vi "Main.vi"(11 "Module Admin":refnum<class "Delacor_lib_QMH_Module Admin.lvclass">) -> ()   [LabVIEW 2021, in "RT Main.lvlib"]
doc: "This template is based off of the Queued Message Handler design pattern and the Queued Message Handler project template that ships with LabVIEW.\n\nThe main difference is that the queue is private to this module and communication between modules is performed via Broadcast and Request events.\n\nRequest events are wrapped in public API methods and are handled in the Event Handling Loop (EHL) of this VI. Any module can register for Broadcast events sent by this module. The EHL generates messages based on user interface actions.\n\nThe Message Handling Loop (MHL) processes messages generated by the EHL, or by other messages. The messages are string values, so new messages can be added easily to the Message Cases case structure in the MHL. Each message cluster can also provide an optional value for Message Data, which is a variant that can be converted to whatever message-specific data is required.\n_____\nBased on DQMH Dev Tools: Project Template 7.1.2.1547."
uses:
  RT Main.lvlib
  <vilib>/Delacor/Delacor QMH/Libraries/Module Admin_class/Delacor_lib_QMH_Module Admin.lvclass
  Module Data--cluster.ctl
  <vilib>/myRIO/Instrument Drivers/Onboard IO/AI/typedefs/AI Reference.ctl
  <vilib>/myRIO/Common/Instrument Driver Framework/Utilities/typedefs/myRIO Generic Hardware Reference.ctl
  <vilib>/myRIO/Common/Instrument Driver Framework/Utilities/typedefs/Hardware Version Enum.ctl
  <vilib>/myRIO/Common/Instrument Driver Framework/Utilities/typedefs/myRIO v1.0 Reference.ctl
  <vilib>/myRIO/Common/Instrument Driver Framework/Utilities/typedefs/Generic FPGA Reference.ctl
  <vilib>/myRIO/Common/Instrument Driver Framework/myRIO v1.0/AI/typedefs/AI Channels List.ctl
  <vilib>/myRIO/Common/Instrument Driver Framework/myRIO v1.0/AI/typedefs/AI Channels Enum.ctl
  <vilib>/myRIO/Common/Instrument Driver Framework/Utilities/typedefs/Analog Scaling Constants List.ctl
  <vilib>/myRIO/Common/Instrument Driver Framework/Utilities/typedefs/Analog Scaling Constants.ctl
  <vilib>/myRIO/Instrument Drivers/Onboard IO/DIO/typedefs/DIO Reference.ctl
  <vilib>/myRIO/Common/Instrument Driver Framework/myRIO v1.0/DIO/typedefs/DIO Channels List.ctl
  <vilib>/myRIO/Common/Instrument Driver Framework/myRIO v1.0/DIO/typedefs/DIO Channels Enum.ctl
  Libraries/Common RT/Modules Launched.ctl
  RT FIFOS--cluster.ctl
  Libraries/Common RT/Hardware Monitoring.ctl
  Hardware Monitoring TL--cluster.ctl
  Stop Argument--cluster.ctl
  <vilib>/Delacor/Delacor QMH/Libraries/Message Queue_class/Delacor_lib_QMH_Message Queue.lvclass/Delacor_lib_QMH_Message Queue.ctl
  <vilib>/Delacor/Delacor QMH/Libraries/Module Admin_class/Delacor_lib_QMH_Module Admin.lvclass/Delacor_lib_QMH_Module Admin.ctl
  Create RT FIFOs Argument--cluster.ctl
  Control Loop Cluster.ctl
  Data Cluster.ctl
  <vilib>/Delacor/Delacor QMH/Libraries/Message Queue_class/Delacor_lib_QMH_Enqueue Message (Single).vi
  <vilib>/Delacor/Delacor QMH/Libraries/Module Admin_class/Delacor_lib_QMH_Get External Launch.vi
  <vilib>/nisyscfg/Close (System).vi
  Timed Loop.vi
  <vilib>/Delacor/Delacor QMH/Libraries/Message Queue_class/Delacor_lib_QMH_Message Queue.lvclass
  Analog Input/Analog Input.lvlib
  <vilib>/myRIO/Instrument Drivers/Onboard IO/AI/AI.lvlib
  Libraries/Common RT/Common RT.lvlib
  <vilib>/nisyscfg/nisyscfg.lvlib
  Digital Inputs/Digital Inputs.lvlib
  <vilib>/myRIO/Instrument Drivers/Onboard IO/DIO/DIO.lvlib
  TDMS/TDMS.lvlib
  RT Interpreter/Manager/RT Interpreter Manager.lvlib
panel:
  out "error out 3":errorcluster
  out "error out 2":errorcluster
  out "error out":errorcluster
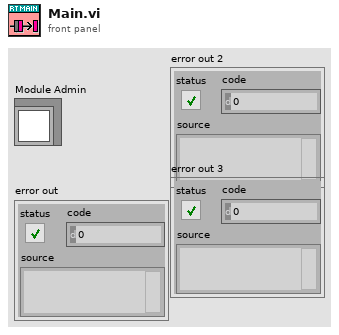
[diagram p1: front panel]
types:
  T1 = typedef "RT Main.lvlib/Request Events--cluster.ctl" = cluster{"Stop Module":refnum<user-event>, "Show Panel":refnum<user-event>, "Hide Panel":refnum<user-event>, "Get Module Execution Status":refnum<user-event>, "Show Diagram":refnum<user-event>, "Private.Launch Control Loop":refnum<user-event>, "Private.RT FIFO Ref":refnum<user-event>, "Private.Create RT FIFOs":refnum<user-event>}
  T2 = typedef "Analog Input.lvlib/Broadcast Events--cluster.ctl" = cluster{"Module Did Init":refnum<user-event>, "Status Updated":refnum<user-event>, "Error Reported":refnum<user-event>, "Module Did Stop":refnum<user-event>, "Update Module Execution Status":refnum<user-event>, "AI Input Reference":refnum<user-event>}
  T3 = typedef "Digital Inputs.lvlib/Broadcast Events--cluster.ctl" = cluster{"Module Did Init":refnum<user-event>, "Status Updated":refnum<user-event>, "Error Reported":refnum<user-event>, "Module Did Stop":refnum<user-event>, "Update Module Execution Status":refnum<user-event>, "Send DI Reference":refnum<user-event>}
  T4 = typedef "TDMS.lvlib/Broadcast Events--cluster.ctl" = cluster{"Module Did Init":refnum<user-event>, "Status Updated":refnum<user-event>, "Error Reported":refnum<user-event>, "Module Did Stop":refnum<user-event>, "Update Module Execution Status":refnum<user-event>}
  T5 = typedef "RT Interpreter Manager.lvlib/Broadcast Events--cluster.ctl" = cluster{"Module Did Init":refnum<user-event>, "Status Updated":refnum<user-event>, "Error Reported":refnum<user-event>, "Module Did Stop":refnum<user-event>, "Update Module Execution Status":refnum<user-event>}
  T6 = typedef "RT Main.lvlib/Hardware Monitoring TL--cluster.ctl" = cluster{"Session in":refnum<k21>, "RT FIFOs--cluster":T7}
  T7 = typedef "RT Main.lvlib/RT FIFOS--cluster.ctl" = cluster{"AIs RT FIFO out":refnum<k33>, "DIOs RT FIFO out":refnum<k33>, "System Status RT FIFO":refnum<k33>}
  T8 = typedef "RT Main.lvlib/Module Data--cluster.ctl" = cluster{"Status":string, "Current Directory":path, "AI Reference":T9, "DIO Reference":T18, "Modules Launched":T21, "RT FIFOs--cluster":T7}
  T9 = typedef "AI.lvlib/AI Reference.ctl" = cluster{"myRIO Reference":T10, "AI Channels List":T14, "AI Scaling Constants List":T16}
  T10 = typedef "myRIO Generic Hardware Reference.ctl" = cluster{"myRIO Model":T11, "myRIO Hardware Reference":T12}
  T11 = typedef "Hardware Version Enum.ctl" = enum16{"Unknown", "myRIO-1900", "myRIO-1950", "roboRIO", "NI ELVIS RIO CM", "ELVIS III"}
  T12 = typedef "myRIO v1.0 Reference.ctl" = cluster{"Generic FPGA Reference":T13, "Allow multiple opens":bool}
  T13 = typedef "Generic FPGA Reference.ctl" = refnum<k20>
  T14 = typedef "AI Channels List.ctl" = T15[]
  T15 = typedef "AI Channels Enum.ctl" = enum16{"Not Connected", "AudioIn/Left", "AudioIn/Right", "C/AI0", "C/AI1", "A/AI0", "A/AI1", "A/AI2", "A/AI3", "A/AI4", "A/AI5", "A/AI6", "A/AI7", "B/AI0", "B/AI1", "B/AI2", "B/AI3", "B/AI4", "B/AI5", "B/AI6", "B/AI7", "AI/AI0", "AI/AI1", "AI/AI2", "AI/AI3", "A/AI0 (DIFF)", "A/AI1 (DIFF)", "A/AI2 (DIFF)", "A/AI3 (DIFF)", "B/AI0 (DIFF)", "B/AI1 (DIFF)", "B/AI2 (DIFF)", "B/AI3 (DIFF)"}
  T16 = typedef "Analog Scaling Constants List.ctl" = T17[]
  T17 = typedef "Analog Scaling Constants.ctl" = cluster{"LSB Weight (Volts)":dbl, "Offset (Volts)":dbl, "Signed?":bool}
  T18 = typedef "DIO.lvlib/DIO Reference.ctl" = cluster{"myRIO Reference":T10, "DIO Channels List":T19}
  T19 = typedef "DIO Channels List.ctl" = T20[]
  T20 = typedef "DIO Channels Enum.ctl" = enum16{"Not Connected", "C/DIO0", "C/DIO1", "C/DIO2", "C/DIO3", "C/DIO4", "C/DIO5", "C/DIO6", "C/DIO7", "A/DIO0", "A/DIO1", "A/DIO2", "A/DIO3", "A/DIO4", "A/DIO5", "A/DIO6", "A/DIO7", "A/DIO8", "A/DIO9", "A/DIO10", "A/DIO11", "A/DIO12", "A/DIO13", "A/DIO14", "A/DIO15", "A/DIO16", "A/DIO17", "A/DIO18", "A/DIO19", "B/DIO0", "B/DIO1", "B/DIO2", "B/DIO3", "B/DIO4", "B/DIO5", "B/DIO6", "B/DIO7", "B/DIO8", "B/DIO9", "B/DIO10", "B/DIO11", "B/DIO12", "B/DIO13", "B/DIO14", "B/DIO15", "B/DIO16", "B/DIO17", "B/DIO18", "B/DIO19", "LED0", "LED1", "LED2", "LED3", "Button0", "DIO/DIO0", "DIO/DIO1", "DIO/DIO2", "DIO/DIO3", "DIO/DIO4", "DIO/DIO5", "DIO/DIO6", "DIO/DIO7", "DIO/DIO8", "DIO/DIO9", "SPI/CS0", "SPI/CS1", "SPI/CS2", "SPI/CS3", "LED RADIO (Green)", "LED RADIO (Red)", "LED COMM (Green)", "LED COMM (Red)", "LED MODE (Green)", "LED MODE (Red)"}
  T21 = typedef "Common RT.lvlib/Modules Launched.ctl" = cluster{"AI Input":bool, "DI Input":bool, "TDMS Module":bool, "UDP Module":bool}
  T22 = enum32{"invalid lock state", "Not Locked", "Locked (No Password)", "Password-protected"}
  T23 = typedef "RT Main.lvlib/Stop Argument--cluster.ctl" = cluster{"Origin":string, "Exit via Stop Module Req?":bool, "Wait for Module to stop?":bool}
  T24 = typedef "RT Main.lvlib/Create RT FIFOs Argument--cluster.ctl" = cluster{"Boolean":bool}
  T25 = typedef "RT Main.lvlib/Control Loop Cluster.ctl" = cluster{"AI Reference":T9, "DIO Reference":T18, "Data Cluster":T26, "TDMS Record?":bool, "Writing?":bool, "RT FIFOs--cluster":T7}
  T26 = typedef "RT Main.lvlib/Data Cluster.ctl" = cluster{"Analog Input":dbl[], "Digital Inputs":bool[], "System Status":T27, "Iteration Duration (ms)":dbl, "Finish Late?":bool}
  T27 = typedef "Common RT.lvlib/Hardware Monitoring.ctl" = cluster{"Memory RAM Free (%)":dbl, "Free Flash memory (%)":dbl, "CPU 0 (%)":u32, "CPU 1 (%)":u32}
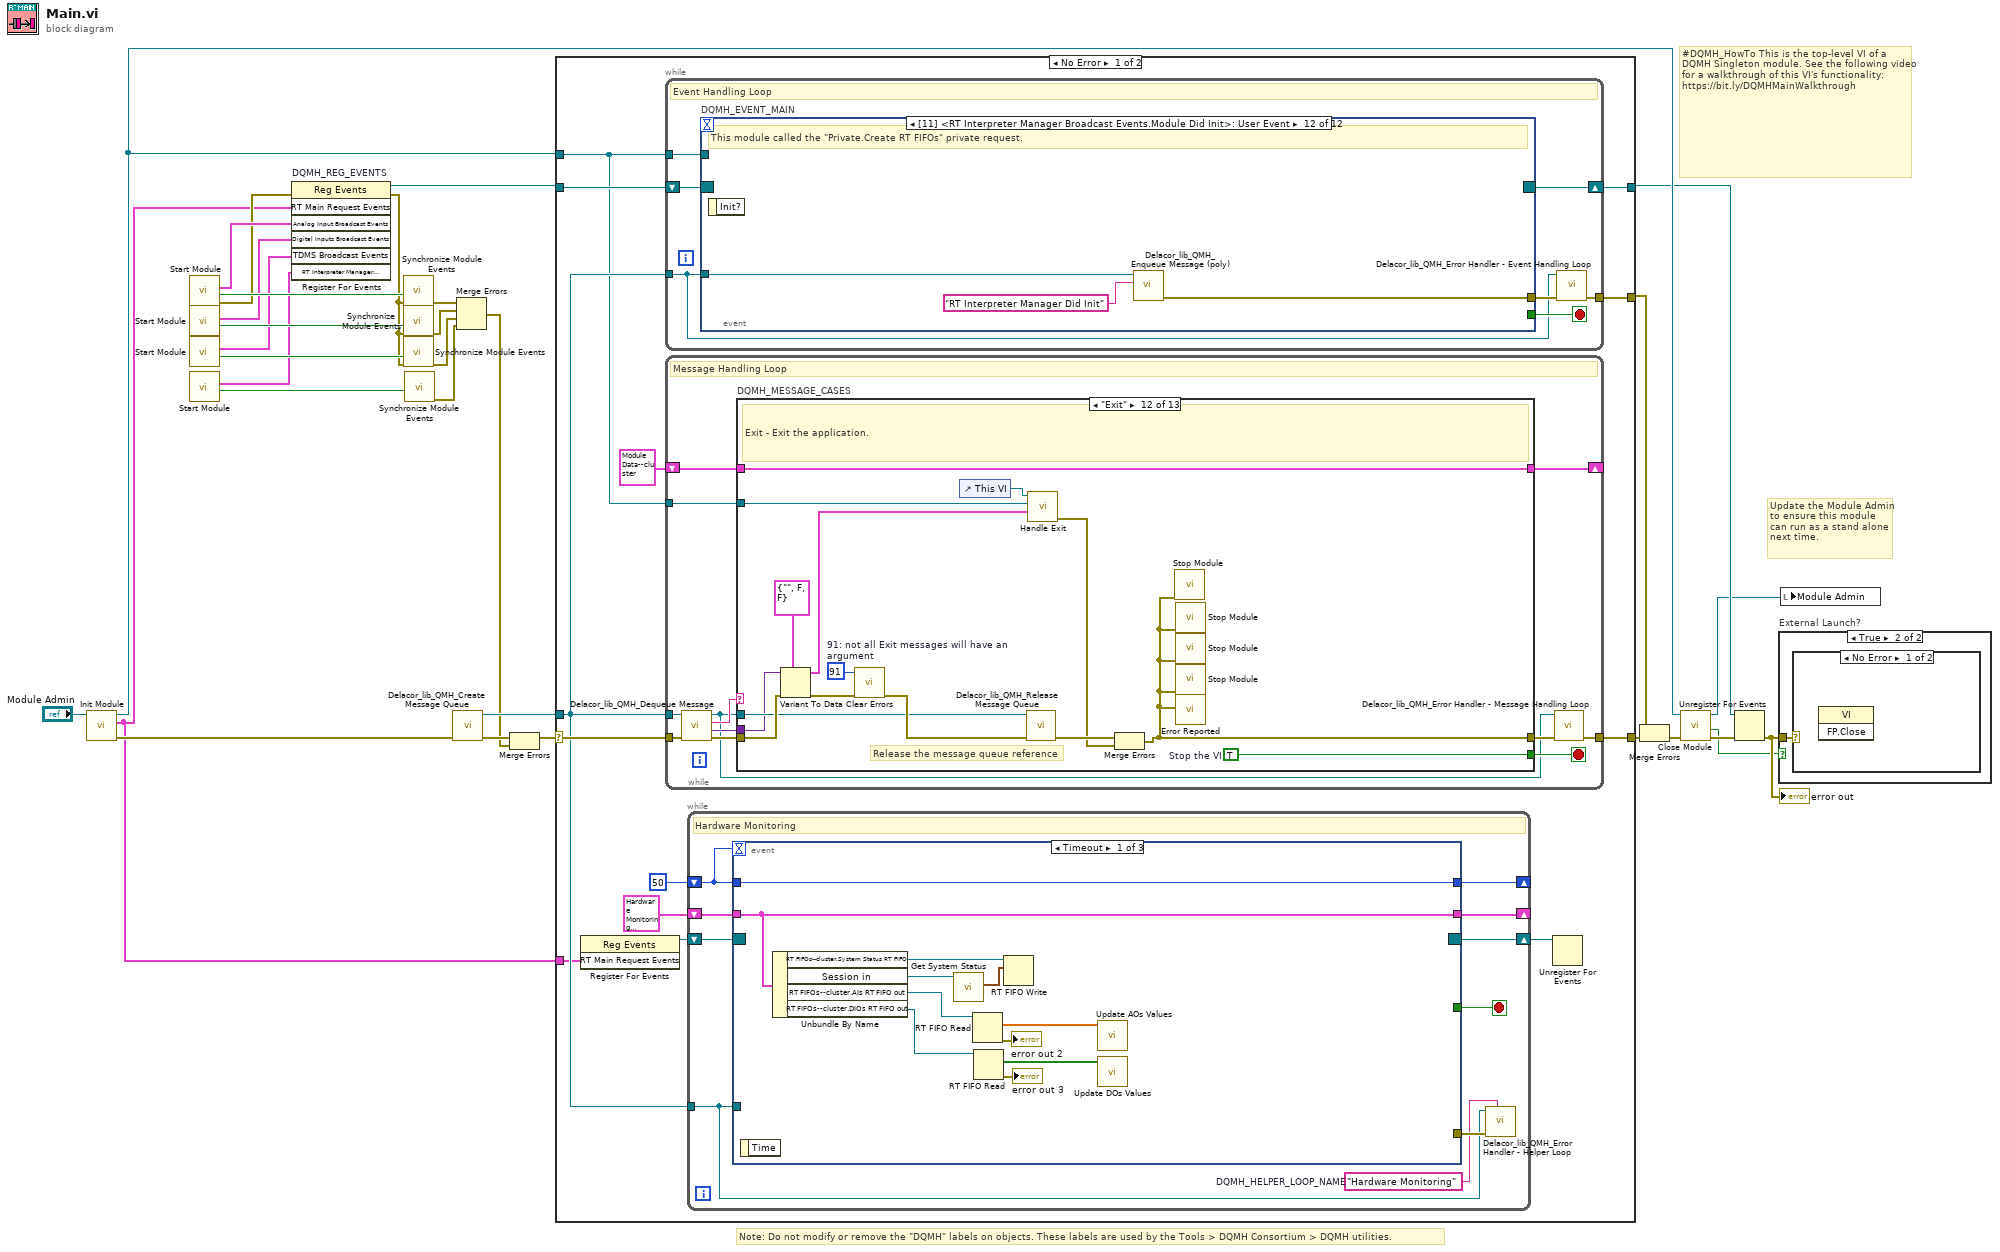
[diagram p0: block diagram]
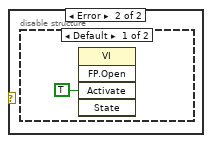
[diagram p3: hidden frame]
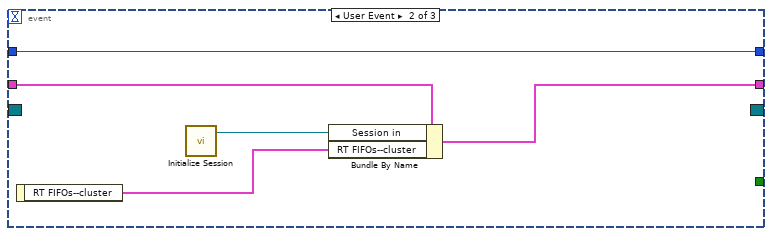
[diagram p5: hidden frame]
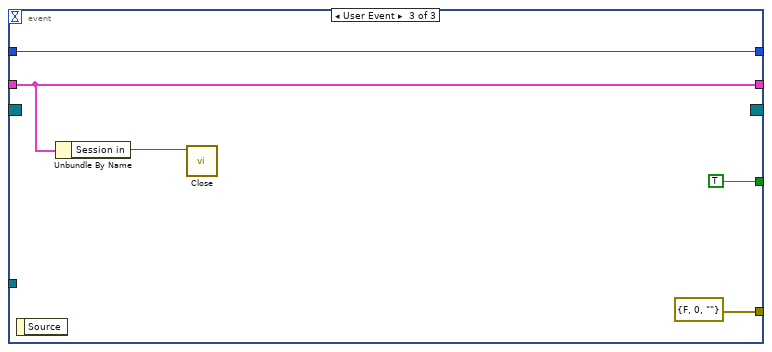
[diagram p6: hidden frame]
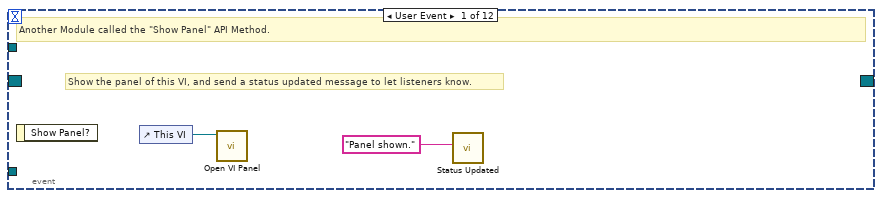
[diagram p7: hidden frame]
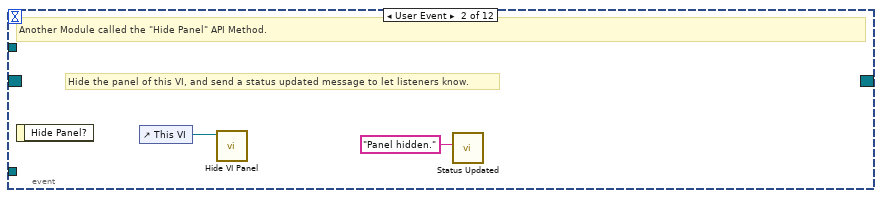
[diagram p8: hidden frame]
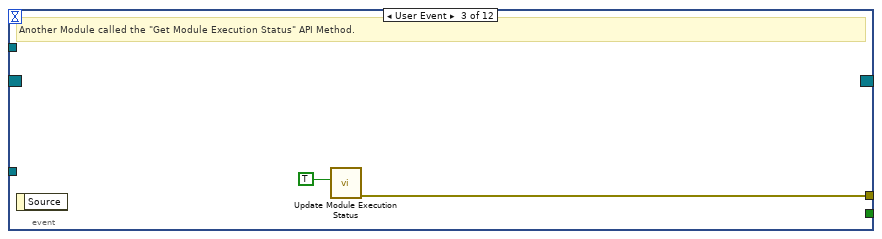
[diagram p9: hidden frame]
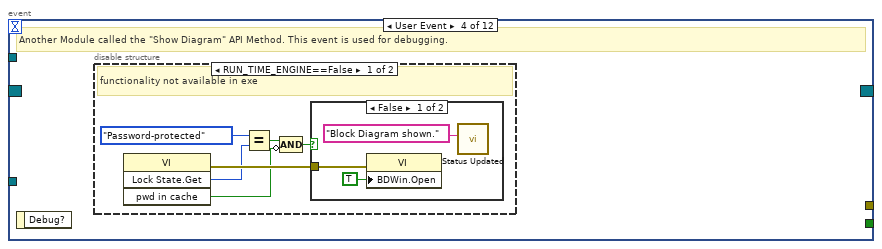
[diagram p10: hidden frame]
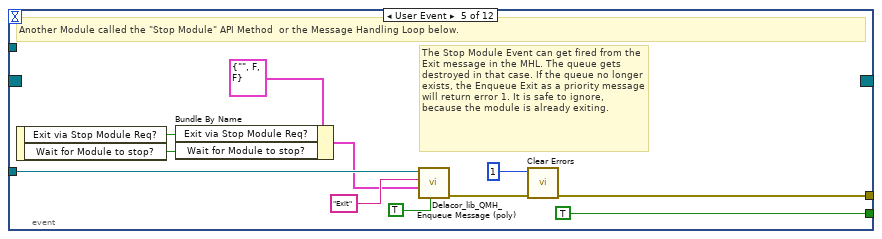
[diagram p13: hidden frame]
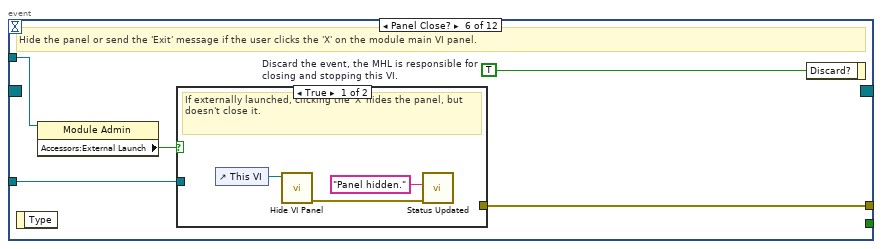
[diagram p14: hidden frame]
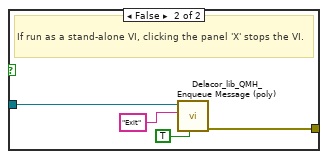
[diagram p15: hidden frame]
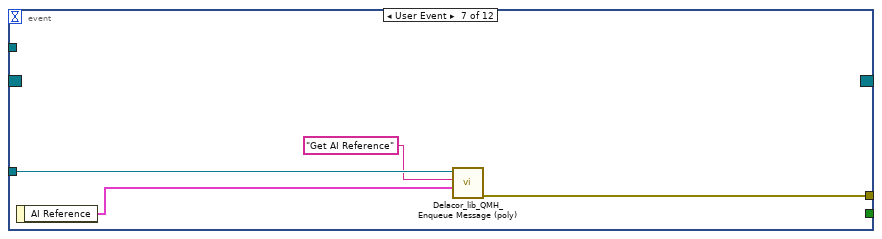
[diagram p16: hidden frame]
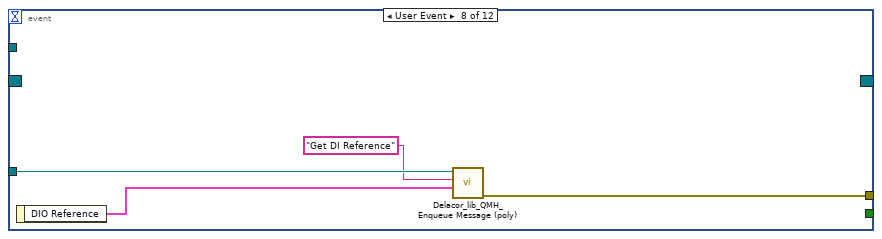
[diagram p17: hidden frame]
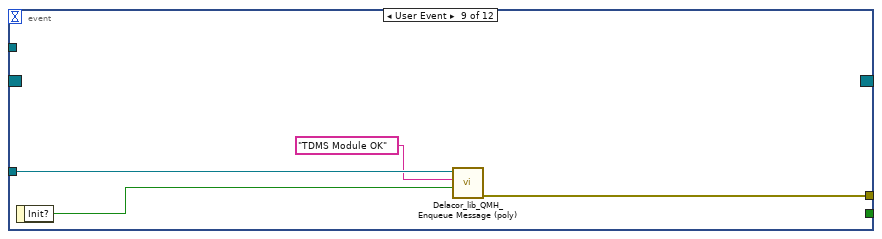
[diagram p18: hidden frame]
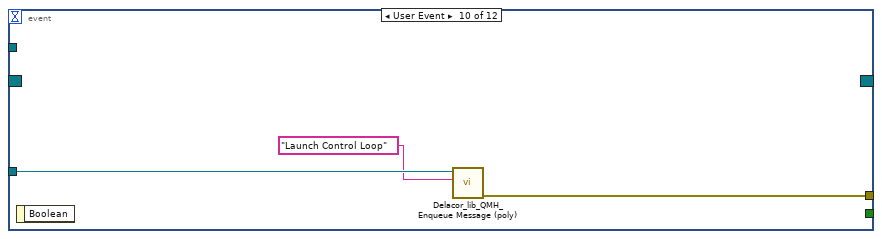
[diagram p19: hidden frame]
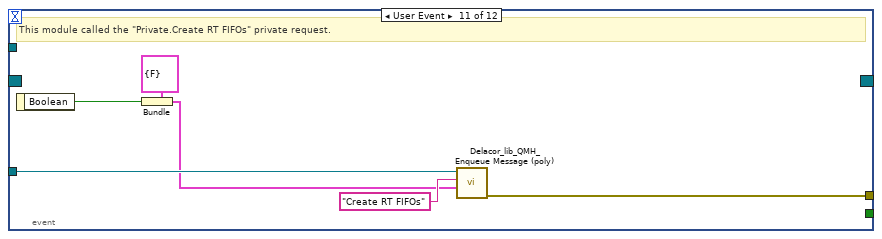
[diagram p20: hidden frame]
diagram:
  # "#DQMH_HowTo This is the top-level VI of a DQMH Singleton module. See the following video for a walkthrough of this VI's functionality: https://bit.ly/DQMHMainWalkthrough"
  # "Note: Do not modify or remove the \"DQMH\" labels on objects. These labels are used by the Tools > DQMH Consortium > DQMH utilities."
  # "Update the Module Admin to ensure this module can run as a stand alone next time."
  n1 = call "Init Module.vi"("Singleton Module Admin in"="Module Admin") -> ("error out"=w30:errorcluster, "RT Main Request Events"=w11:T1, "Singleton Module Admin out"=w23:refnum<class "Delacor_lib_QMH_Module Admin.lvclass">)  [unwired: 8 in]
  n2 = call "Start Module.vi"() -> ("error out"=w14:errorcluster, "Wait for Event Sync?"=w15:bool, "Analog Input Broadcast Events"=w16:T2)  [unwired: 7 in, 2 out]
  n3 = call "Start Module.vi"() -> ("Wait for Event Sync?"=w10:bool, "Digital Inputs Broadcast Events"=w9:T3)  [unwired: 7 in, 3 out]
  n4 = call "Start Module.vi"() -> ("Wait for Event Sync?"=w6:bool, "TDMS Broadcast Events"=w7:T4)  [unwired: 8 in, 2 out]
  n5 = call "Start Module.vi"() -> ("Wait for Event Sync?"=w1:bool, "RT Interpreter Manager Broadcast Events"=w2:T5)  [unwired: 7 in, 3 out]
  n6 = register-events "DQMH_REG_EVENTS"(error in=w14, w11, w16, w9, w7, w2) -> (reference out=w21:refnum<event-registration>, error out=w4:errorcluster)  [unwired: 1 in]
  n7 = call "Synchronize Module Events.vi"("error in"=w4, "Wait for Event Sync?"=w15) -> ("error out"=w13:errorcluster)  [unwired: 9 in]
  n8 = call "Synchronize Module Events.vi"("error in"=w4, "Wait for Event Sync?"=w10) -> ("error out"=w8:errorcluster)  [unwired: 9 in]
  n9 = call "Synchronize Module Events.vi"("error in"=w4, "Wait for Event Sync?"=w6) -> ("error out"=w5:errorcluster)  [unwired: 9 in]
  n10 = call "Synchronize Module Events.vi"("Wait for Event Sync?"=w1) -> ("error out"=w3:errorcluster)  [unwired: 10 in]
  n11 = call <vilib>:"Delacor_lib_QMH_Create Message Queue.vi"("error in"=w30) -> ("error out"=w25:errorcluster, "Message Queue"=w20:refnum<class "Delacor_lib_QMH_Message Queue.lvclass">)  [unwired: 9 in]
  n12 = Merge Errors(w13, w8, w5, w3) -> (w12:errorcluster)
  n13 = Merge Errors(w25, w12) -> (w24:errorcluster)
  n14 = case shown="No Error" w24 {
    selector: w24 -> [w42 w296]
    tunnel: [w44 w295] -> w31
    tunnel: [w41 w294] -> w22
    tunnel: w21 -> [w39 w294]
    tunnel: w20 -> [w38 w289]
    tunnel: [w43 _] -> w28
    tunnel: w23 -> [w37 w290]
    tunnel: w11 -> [w36 _]
    frame No Error {
      n15 = register-events ("DQMH_HELPER_REGFOREVENTS")(w36) -> (reference out=w34:refnum<event-registration>)  [unwired: 2 in, 1 out]
      n16 = while {
        tunnel: w38 -> [w76]
        shift-right: [w79] -> w41
        shift-left: w39 -> [w80]
        tunnel: [w81] -> w43
        tunnel: w37 -> [w77]
        stop <- w78 stop-if-true
        # "Event Handling Loop"
        n17 = event "DQMH_EVENT_MAIN" shown="[11] <RT Interpreter Manager Broadcast Events.Module Did Init>: User Event" {
          selector: w80 -> [_ _ _ _ _ _ _ _ _ _ _ _]
          dyn-events: [_ _ _ _ _ _ _ _ _ _ _ _] -> w79
          timeout: _ -> [_ _ _ _ _ _ _ _ _ _ _ _]
          tunnel: [_ _ _ _ TRUE ("Discard?") _ _ _ _ _ _ _] -> w78
          tunnel: w76 -> [_ _ _ _ w104 w111 w124 w128 w132 w135 w141 w144]
          tunnel: [_ _ w88 _ w107 w113 w121 w125 w129 w133 w136 w142] -> w82
          tunnel: w77 -> [_ _ _ _ _ w110 _ _ _ _ _ _]
          event User Event {
            # "Show the panel of this VI, and send a status updated message to let listeners know."
            # "Another Module called the \"Show Panel\" API Method."
            n18 = event-data() -> ()  [unwired: 1 in, 1 out]
            n19 = control-ref of="This VI"() -> (w84:refnum<vi>)
            n20 = call "Open VI Panel.vi"("VI"=w84) -> ()  [unwired: 10 in, 1 out]
            n21 = call "Status Updated.vi"("Status"="Panel shown." ("format string")) -> ()  [unwired: 10 in, 1 out]
          }
          event User Event {
            # "Hide the panel of this VI, and send a status updated message to let listeners know."
            # "Another Module called the \"Hide Panel\" API Method."
            n22 = event-data() -> ()  [unwired: 1 in, 1 out]
            n23 = control-ref of="This VI"() -> (w86:refnum<vi>)
            n24 = call "Hide VI Panel.vi"("VI"=w86) -> ()  [unwired: 10 in, 1 out]
            n25 = call "Status Updated.vi"("Status"="Panel hidden." ("format string")) -> ()  [unwired: 10 in, 1 out]
          }
          event User Event {
            # "Another Module called the \"Get Module Execution Status\" API Method."
            n26 = event-data() -> ()  [unwired: 1 in, 1 out]
            n27 = call "Update Module Execution Status.vi"("Running?"=TRUE) -> ("error out"=w88:errorcluster)  [unwired: 10 in]
          }
          event User Event {
            # "Another Module called the \"Show Diagram\" API Method. This event is used for debugging."
            n28 = event-data() -> ()  [unwired: 1 in, 1 out]
            n29 = disable-structure shown="RUN_TIME_ENGINE==False" {
              frame condition #0 (active) {
                # "functionality not available in exe"
                n30 = invoke on="Invoke Node" class="VI" method="Lock State.Get"() -> (error out=w94:errorcluster, "Get Lock State"=w93:T22, "pwd in cache"=w90:bool)  [unwired: 4 in, 1 out]
                n31 = Equal?(x=T22."Password-protected", y=w93) -> (x = y?=w91:bool)
                n32 = Compound Arithmetic op=AND(w91, invert w90) -> (w89:bool)
                n33 = case shown="False" w89 {
                  tunnel: w94 -> [w97 _]
                  frame False {
                    n34 = property on="Property Node" class="VI"(error in=w97, "BDWin.Open"=TRUE ("Block Diagram Window:Open")) -> ()  [unwired: 1 in, 2 out]
                    n35 = call "Status Updated.vi"("Status"="Block Diagram shown." ("format string")) -> ()  [unwired: 10 in, 1 out]
                  }
                  frame True {
                    # "Password-protected VI, and the password is not in the cache. Do not show the diagram."
                  }
                }
              }
              frame condition #1 {
              }
            }
          }
          event User Event {
            # "The Stop Module Event can get fired from the Exit message in the MHL. The queue gets destroyed in that case. If the queue no longer exists, the Enqueue Exit as a priority message will return error 1. It is safe to ignore, because the module is already exiting."
            # "Another Module called the \"Stop Module\" API Method  or the Message Handling Loop below."
            n36 = event-data() -> ("Exit via Stop Module Req?"=w100:bool, "Wait for Module to stop?"=w99:bool)  [unwired: 1 in]
            n37 = Bundle By Name(cluster=T23 {"Origin"="", "Exit via Stop Module Req?"=FALSE, "Wait for Module to stop?"=FALSE} ("Stop Argument"), "Exit via Stop Module Req?"=w100, "Wait for Module to stop?"=w99) -> (w98:T23)
            n38 = call-poly <vilib>:"Delacor_lib_QMH_Enqueue Message (poly).vi"("Priority Message? (F)"=TRUE, "Message Data"=w98, "Message"="Exit", "Message Queue in"=w104) -> ("error out"=w108:errorcluster)  [unwired: 6 in, 1 out]
            n39 = call <vilib>:"Clear Errors.vi"("error in (no error)"=w108, "specific error code to clear (0: all)"=1) -> ("error out"=w107:errorcluster)  [unwired: 4 in, 1 out]
          }
          event Panel Close? {
            w112 = TRUE  # Discard the event, the MHL is responsible for closing and stopping this VI.
            # "Hide the panel or send the 'Exit' message if the user clicks the 'X' on the module main VI panel."
            n40 = event-data() -> ()  [unwired: 1 in, 1 out]
            n41 = property on="Property Node" class="Module Admin"(reference=w110) -> ("Accessors:External Launch"=w109:bool)  [unwired: 1 in, 2 out]
            n42 = case shown="True" w109 {
              tunnel: w111 -> [_ w119]
              tunnel: [_ w120] -> w113
              frame True {
                # "If externally launched, clicking the 'X' hides the panel, but doesn't close it."
                n43 = control-ref of="This VI"() -> (w116:refnum<vi>)
                n44 = call "Hide VI Panel.vi"("VI"=w116) -> ("error out"=w114:errorcluster)  [unwired: 10 in]
                n45 = call "Status Updated.vi"("error in"=w114, "Status"="Panel hidden." ("format string")) -> ()  [unwired: 9 in, 1 out]
              }
              frame False {
                # "If run as a stand-alone VI, clicking the panel 'X' stops the VI."
                n46 = call-poly <vilib>:"Delacor_lib_QMH_Enqueue Message (poly).vi"("Priority Message? (F)"=TRUE, "Message"="Exit", "Message Queue in"=w119) -> ("error out"=w120:errorcluster)  [unwired: 7 in, 1 out]
              }
            }
            n47 = event-data ("Event Filter Node")("Discard?"=w112) -> ()  [unwired: 1 in, 1 out]
          }
          event User Event {
            n48 = event-data() -> ("AI Reference"=w122:T9)  [unwired: 1 in]
            n49 = call-poly <vilib>:"Delacor_lib_QMH_Enqueue Message (poly).vi"("Message Data"=w122, "Message"="Get AI Reference", "Message Queue in"=w124) -> ("error out"=w121:errorcluster)  [unwired: 7 in, 1 out]
          }
          event User Event {
            n50 = event-data() -> ("DIO Reference"=w126:T18)  [unwired: 1 in]
            n51 = call-poly <vilib>:"Delacor_lib_QMH_Enqueue Message (poly).vi"("Message Data"=w126, "Message"="Get DI Reference", "Message Queue in"=w128) -> ("error out"=w125:errorcluster)  [unwired: 7 in, 1 out]
          }
          event User Event {
            n52 = event-data() -> ("Init?"=w130:bool)  [unwired: 1 in]
            n53 = call-poly <vilib>:"Delacor_lib_QMH_Enqueue Message (poly).vi"("Message Data"=w130, "Message"="TDMS Module OK", "Message Queue in"=w132) -> ("error out"=w129:errorcluster)  [unwired: 7 in, 1 out]
          }
          event User Event {
            n54 = event-data() -> ()  [unwired: 1 in, 1 out]
            n55 = call-poly <vilib>:"Delacor_lib_QMH_Enqueue Message (poly).vi"("Message"="Launch Control Loop", "Message Queue in"=w135) -> ("error out"=w133:errorcluster)  [unwired: 8 in, 1 out]
          }
          event User Event {
            # "This module called the \"Private.Create RT FIFOs\" private request."
            n56 = event-data() -> ("Boolean"=w137:bool)  [unwired: 1 in]
            n57 = Bundle(cluster=T24 {"Boolean"=FALSE} ("Create RT FIFOs Argument"), "Boolean"=w137) -> (w138:T24)
            n58 = call-poly <vilib>:"Delacor_lib_QMH_Enqueue Message (poly).vi"("Message Data"=w138, "Message"="Create RT FIFOs", "Message Queue in"=w141) -> ("error out"=w136:errorcluster)  [unwired: 7 in, 1 out]
          }
          event User Event {
            # "This module called the \"Private.Create RT FIFOs\" private request."
            n59 = event-data() -> ()  [unwired: 1 in, 1 out]
            n60 = call-poly <vilib>:"Delacor_lib_QMH_Enqueue Message (poly).vi"("Message"="RT Interpreter Manager Did Init", "Message Queue in"=w144) -> ("error out"=w142:errorcluster)  [unwired: 8 in, 1 out]
          }
        }
        n61 = call-dynamic "Delacor_lib_QMH_Error Handler - Event Handling Loop.vi"("error in"=w82, "Message Queue in"=w76) -> ("dup error in"=w81:errorcluster)  [unwired: 8 in, 1 out]
      }
      n62 = while {
        tunnel: w38 -> [w145]
        shift-right: [w153] -> _
        shift-left: T8 {"Status"="", "Current Directory"=path "", "AI Reference"={"myRIO Reference"={"myRIO Model"=enum."Unknown", "myRIO Hardware Reference"={"Generic FPGA Reference"=refnum, "Allow multiple opens"=FALSE}}, "AI Channels List"=[], "AI Scaling Constants List"=[]}, "DIO Reference"={"myRIO Reference"={"myRIO Model"=enum."Unknown", "myRIO Hardware Reference"={"Generic FPGA Reference"=refnum, "Allow multiple opens"=FALSE}}, "DIO Channels List"=[]}, "Modules Launched"={"AI Input"=FALSE, "DI Input"=FALSE, "TDMS Module"=FALSE, "UDP Module"=FALSE}, "RT FIFOs--cluster"={"AIs RT FIFO out"=refnum, "DIOs RT FIFO out"=refnum, "System Status RT FIFO"=refnum}} ("Data Cluster") -> [w154]
        tunnel: w42 -> [w156]
        tunnel: [w148] -> w44
        tunnel: w37 -> [w149]
        stop <- w152 stop-if-true
        # "Message Handling Loop"
        n63 = call-dynamic "Delacor_lib_QMH_Dequeue Message.vi"("error in"=w156, "Message Queue in"=w145) -> ("error out"=w155:errorcluster, "Message Data"=w150:variant, "Message"=w151:string, "Message Queue out"=w146:refnum<class "Delacor_lib_QMH_Message Queue.lvclass">)  [unwired: 6 in]
        n64 = case "DQMH_MESSAGE_CASES" shown="\"Exit\"" w151 {
          selector: w151 -> [_ _ _ _ _ _ _ _ _ _ _ _ w284]
          tunnel: w146 -> [_ _ _ _ _ _ _ _ _ _ w250 w273 _]
          tunnel: w155 -> [w167 w169 w181 w196 w207 w218 w229 w240 w244 w246 w257 w278 w287]
          tunnel: [w158 w169 w170 w187 w200 w211 w230 w237 w243 w246 w253 w264 w288] -> w147
          tunnel: w154 -> [w159 w168 w176 w193 w205 w216 w235 w241 w242 w245 w252 w272 w285]
          tunnel: [w160 w168 w175 w192 w204 w215 w235 w238 w242 w245 w252 w272 w285] -> w153
          tunnel: [_ _ _ _ _ _ _ _ _ _ _ w271 _] -> w152
          tunnel: w150 -> [_ _ w180 w195 _ _ _ _ _ _ w251 w270 _]
          tunnel: w149 -> [w165 _ _ _ _ _ _ _ _ _ w249 w265 _]
          frame "Initialize" {
            # "Initialize - Any operation that needs to be done before the module can receive messages. Synchronize Caller Events.vi will inform Start Module.vi that the module has launched and is ready to receive messages. Module Did Init.vi will broadcast that the module initialized."
            n65 = call "Synchronize Caller Events.vi"("error in"=w167, "Singleton Module Admin in"=w165) -> ("error out"=w166:errorcluster)  [unwired: 8 in, 1 out]
            n66 = call "Module Name--constant.vi"() -> ("Module Name"=w163:string)  [unwired: 11 in]
            n67 = call "Module Did Init.vi"("error in"=w166, "Initialized?"=TRUE, "Origin"=w163) -> ("error out"=w157:errorcluster)  [unwired: 8 in]
            n68 = Current VI's Path() -> (path=w162:path)
            n69 = Strip Path(path=w162) -> (stripped path=w161:path)  [unwired: 1 out]
            n70 = Bundle By Name(cluster=w159, "Current Directory"=w161) -> (w160:T8)
            n71 = call "Create RT FIFOs.vi"("error in"=w157) -> ("error out"=w158:errorcluster)  [unwired: 10 in]
          }
          frame "---Module Specific---" {
            # "Separator -- The following cases handle messages specific to this Module."
          }
          frame "Get AI Reference" {
            # "Get AI Reference"
            n72 = Variant To Data(error in=w181, type=T9 {"myRIO Reference"={"myRIO Model"=enum."Unknown", "myRIO Hardware Reference"={"Generic FPGA Reference"=refnum, "Allow multiple opens"=FALSE}}, "AI Channels List"=[], "AI Scaling Constants List"=[]} ("AI Reference"), Variant=w180) -> (data=w178:T9, error out=w171:errorcluster)
            n73 = Bundle By Name(cluster=w176, "Modules Launched.AI Input"=TRUE, "AI Reference"=w178) -> (w175:T8)
            n74 = Unbundle By Name(w175) -> ("Modules Launched"=w174:T21)
            n75 = Cluster To Array(cluster=w174) -> (array=w173:bool[])
            n76 = And Array Elements(Boolean array=w173) -> (logical AND=w172:bool)
            n77 = case shown="True" w172 {
              tunnel: w171 -> [w182 w183]
              tunnel: [w182 w184] -> w170
              frame False {
              }
              frame True {
                n78 = call "Launch Control Loop.vi"("error in"=w183) -> ("error out"=w184:errorcluster)  [unwired: 10 in]
              }
            }
          }
          frame "Get DI Reference" {
            # "Get DI Reference"
            n79 = Variant To Data(error in=w196, type=T18 {"myRIO Reference"={"myRIO Model"=enum."Unknown", "myRIO Hardware Reference"={"Generic FPGA Reference"=refnum, "Allow multiple opens"=FALSE}}, "DIO Channels List"=[]} ("DIO Ref Out"), Variant=w195) -> (data=w185:T18, error out=w188:errorcluster)
            n80 = Bundle By Name(cluster=w193, "Modules Launched.DI Input"=TRUE ("Modules Launched.AI Input"), "DIO Reference"=w185) -> (w192:T8)
            n81 = Unbundle By Name(w192) -> ("Modules Launched"=w191:T21)
            n82 = Cluster To Array(cluster=w191) -> (array=w190:bool[])
            n83 = And Array Elements(Boolean array=w190) -> (logical AND=w189:bool)
            n84 = case shown="True" w189 {
              tunnel: w188 -> [w197 w198]
              tunnel: [w197 w199] -> w187
              frame False {
              }
              frame True {
                n85 = call "Launch Control Loop.vi"("error in"=w198) -> ("error out"=w199:errorcluster)  [unwired: 10 in]
              }
            }
          }
          frame "RT Interpreter Manager Did Init" {
            # "Get DI Reference"
            n86 = Bundle By Name(cluster=w205, "Modules Launched.UDP Module"=TRUE ("Modules Launched.AI Input")) -> (w204:T8)
            n87 = Unbundle By Name(w204) -> ("Modules Launched"=w203:T21)
            n88 = Cluster To Array(cluster=w203) -> (array=w202:bool[])
            n89 = And Array Elements(Boolean array=w202) -> (logical AND=w201:bool)
            n90 = case shown="True" w201 {
              tunnel: w207 -> [w208 w209]
              tunnel: [w208 w210] -> w200
              frame False {
              }
              frame True {
                n91 = call "Launch Control Loop.vi"("error in"=w209) -> ("error out"=w210:errorcluster)  [unwired: 10 in]
              }
            }
          }
          frame "TDMS Module OK" {
            # "TDMS Module OK"
            n92 = Bundle By Name(cluster=w216, "Modules Launched.TDMS Module"=TRUE ("Modules Launched.AI Input")) -> (w215:T8)
            n93 = Unbundle By Name(w215) -> ("Modules Launched"=w214:T21)
            n94 = Cluster To Array(cluster=w214) -> (array=w213:bool[])
            n95 = And Array Elements(Boolean array=w213) -> (logical AND=w212:bool)
            n96 = case shown="True" w212 {
              tunnel: w218 -> [w219 w220]
              tunnel: [w219 w221] -> w211
              frame False {
              }
              frame True {
                n97 = call "Launch Control Loop.vi"("error in"=w220) -> ("error out"=w221:errorcluster)  [unwired: 10 in]
              }
            }
          }
          frame "Launch Control Loop" {
            # "Launch Control Loop"
            n98 = Unbundle By Name(w235) -> ("AI Reference"=w233:T9, "DIO Reference"=w226:T18, "RT FIFOs--cluster"=w225:T7)
            n99 = vi-ref "RT Main.lvlib:Timed Loop.vi"() -> (w223:refnum<vi>)
            n100 = property class="VI Interface Type 0"(reference=w223) -> ("Name"=w222:string)  [unwired: 1 in, 2 out]
            n101 = Bundle By Name(cluster=T25 {"AI Reference"={"myRIO Reference"={"myRIO Model"=enum."Unknown", "myRIO Hardware Reference"={"Generic FPGA Reference"=refnum, "Allow multiple opens"=FALSE}}, "AI Channels List"=[], "AI Scaling Constants List"=[]}, "DIO Reference"={"myRIO Reference"={"myRIO Model"=enum."Unknown", "myRIO Hardware Reference"={"Generic FPGA Reference"=refnum, "Allow multiple opens"=FALSE}}, "DIO Channels List"=[]}, "Data Cluster"={"Analog Input"=[], "Digital Inputs"=[], "System Status"={"Memory RAM Free (%)"=0.0, "Free Flash memory (%)"=0.0, "CPU 0 (%)"=0, "CPU 1 (%)"=0}, "Iteration Duration (ms)"=0.0, "Finish Late?"=FALSE}, "TDMS Record?"=FALSE, "Writing?"=FALSE, "RT FIFOs--cluster"={"AIs RT FIFO out"=refnum, "DIOs RT FIFO out"=refnum, "System Status RT FIFO"=refnum}} ("Control Loop Cluster"), "AI Reference"=w233, "DIO Reference"=w226, "RT FIFOs--cluster"=w225) -> (w231:T25)
            n102 = Open VI Reference(type specifier VI Refnum (for type only)=refnum<vi> refnum, vi path=w222, options=128, error in (no error)=w229) -> (vi reference=w228:refnum<vi>, error out=w232:errorcluster)  [unwired: 2 in]
            n103 = call-by-ref "Start Asynchronous Call"(reference=w228, error in=w232, "Control Loop Cluster"=w231) -> (error out=w230:errorcluster)  [unwired: 10 in, 2 out]
          }
          frame "Create RT FIFOs" {
            n104 = call "Create all RT FIFOS.vi"("error in"=w240) -> ("error out"=w239:errorcluster, "RT FIFOs--cluster"=w236:T7)  [unwired: 9 in]
            n105 = Bundle By Name(cluster=w241, "RT FIFOs--cluster"=w236) -> (w238:T8)
            n106 = call "Get RT FIFO HW Ref.vi"("error in"=w239, "RT FIFOs--cluster"=w236) -> ("error out"=w237:errorcluster)  [unwired: 9 in]
          }
          frame "---Copy This Frame---" {
            # "Duplicate this frame when creating new messages.  Change this comment in the duplicated frame to describe this message."
            n107 = Merge Errors(w244) -> (w243:errorcluster)
          }
          frame "---Exit and Error Handling---" {
            # "Separator - The following cases handle errors and exit messages."
          }
          frame "Error" {
            # "#DQMH_CodeRecommended - If the module is running in standalone mode (External Launch = FALSE), this code will pop up an error dialog and call the 'Exit' message if an error occurs. Add more fine-grained error management here."
            # "Error - Check the error message data and respond accordingly. This message is sent by the \"Error Handler\" VIs at the end of each loop in this application."
            n108 = property on="Property Node" class="Module Admin"(reference=w249) -> ("Accessors:External Launch"=w248:bool)  [unwired: 1 in, 2 out]
            n109 = Variant To Data(error in=w257, type=errorcluster {"status"=FALSE, "code"=0, "source"=""} ("error constant"), Variant=w251) -> (data=w247:errorcluster, error out=w255:errorcluster)
            n110 = local write "error out"(w247) -> ()
            n111 = call "Error Reported.vi"("Error"=w247) -> ()  [unwired: 10 in, 1 out]
            n112 = case shown="False" w248 {
              tunnel: [w262 _] -> w254
              tunnel: w250 -> [w260 _]
              tunnel: w247 -> [w261 _]
              frame False {
                n113 = disable-structure shown="DQMH_Disable_SEH==TRUE" {
                  disable-tunnel: w261 -> [w263 _]
                  frame condition #0 (active) {
                    # "If the module is running standalone, then pop up an error dialog and call the \"Exit\" message."
                    n114 = call <vilib>:"Simple Error Handler.vi"("error in (no error)"=w263) -> ()  [unwired: 4 in, 5 out]
                  }
                  frame condition #1 {
                    # "To prevent the Simple Error Handler VI from being loaded (e.g. when deploying to a Real-Time target), add the Conditional Disable Symbol \"DQMH_Disable_SEH\" to your project and set it to TRUE."
                  }
                }
                n115 = call-poly <vilib>:"Delacor_lib_QMH_Enqueue Message (poly).vi"("Priority Message? (F)"=TRUE, "Message"="Exit", "Message Queue in"=w260) -> ("error out"=w262:errorcluster)  [unwired: 7 in, 1 out]
              }
              frame True {
                # "If the module was launched externally, calling the Error Reported broadcast VI is the only action performed by the \"Error\" message. The module's caller can then process the error appropriately."
              }
            }
            n116 = Merge Errors(w255, w254) -> (w253:errorcluster)
          }
          frame "Exit" {
            w269 = 91  # 91: not all Exit messages will have an argument
            w271 = TRUE  # Stop the VI
            # "Release the message queue reference"
            # "Exit - Exit the application."
            n117 = Variant To Data(error in=w278, type=T23 {"Origin"="", "Exit via Stop Module Req?"=FALSE, "Wait for Module to stop?"=FALSE} ("Stop Argument"), Variant=w270) -> (data=w267:T23, error out=w275:errorcluster)
            n118 = call <vilib>:"Clear Errors.vi"("error in (no error)"=w275, "specific error code to clear (0: all)"=w269) -> ("error out"=w277:errorcluster)  [unwired: 4 in, 1 out]
            n119 = control-ref of="This VI"() -> (w266:refnum<vi>)
            n120 = call-dynamic "Delacor_lib_QMH_Release Message Queue.vi"("error in"=w277, "Message Queue"=w273) -> ("error out"=w276:errorcluster)  [unwired: 9 in]
            n121 = call "Handle Exit.vi"("Stop Argument"=w267, "Admin in"=w265, "VI reference"=w266) -> ("error out"=w274:errorcluster)  [unwired: 7 in, 1 out]
            n122 = Merge Errors(w276, w274) -> (w264:errorcluster)
            n123 = call "Stop Module.vi"("error in"=w264) -> ()  [unwired: 10 in, 1 out]
            n124 = call "Stop Module.vi"("error in"=w264) -> ()  [unwired: 10 in, 1 out]
            n125 = call "Stop Module.vi"("error in"=w264) -> ()  [unwired: 10 in, 1 out]
            n126 = call "Stop Module.vi"("error in"=w264) -> ()  [unwired: 10 in, 1 out]
            n127 = call "Error Reported.vi"("Error"=w264) -> ()  [unwired: 10 in, 1 out]
          }
          frame Default {
            # "'Default' case only runs if there is a message that isn't defined in any of the other cases.  Output a programming error."
            n128 = call "Module Name--constant.vi"() -> ("Module Name"=w283:string)  [unwired: 11 in]
            n129 = Format Into String(format string="The invalid message string \"%s\" was received in the Message Handling Loop for module \"%s\".", w284, w283) -> (resulting string=w279:string)  [unwired: 2 in, 1 out]
            n130 = call <vilib>:"Error Cluster From Error Code.vi"("show call chain? (False)"=TRUE, "error message (\"\")"=w279, "error code (0)"=1) -> ("error out"=w286:errorcluster)  [unwired: 6 in]
            n131 = Merge Errors(w287, w286) -> (w288:errorcluster)
          }
        }
        n132 = call-dynamic "Delacor_lib_QMH_Error Handler - Message Handling Loop.vi"("error in"=w147, "Message Queue in"=w146) -> ("dup error in"=w148:errorcluster)  [unwired: 8 in, 1 out]
      }
      n133 = while "DQMH_HELPER_LOOP" {
        shift-right: [w54] -> _
        shift-left: 50 -> [w53]
        shift-right: [w51] -> w35
        shift-left: w34 -> [w52]
        tunnel: w38 -> [w48]
        shift-right: [w45] -> _
        shift-left: T6 {"Session in"="localhost", "RT FIFOs--cluster"={"AIs RT FIFO out"=refnum, "DIOs RT FIFO out"=refnum, "System Status RT FIFO"=refnum}} ("Hardware Monitoring TL--cluster.ctl") -> [w46]
        stop <- w50 stop-if-true
        w47 = "Hardware Monitoring"  # DQMH_HELPER_LOOP_NAME
        # "Hardware Monitoring"
        n134 = event "DQMH_HELPER_EVENT_STRUCTURE" shown="[0] Timeout" {
          selector: w52 -> [_ _ _]
          dyn-events: [_ _ _] -> w51
          timeout: w53 -> [_ _ _]
          tunnel: w53 -> [w65 w70 w75]
          tunnel: [w65 w70 w75] -> w54
          tunnel: [_ _ TRUE] -> w50
          tunnel: [_ _ errorcluster {"status"=FALSE, "code"=0, "source"=""} ("error constant")] -> w49
          tunnel: w48 -> [_ _ _]
          tunnel: w46 -> [w64 w69 w72]
          tunnel: [w64 w66 w72] -> w45
          event Timeout {
            n135 = event-data() -> ()  [unwired: 1 in, 1 out]
            n136 = Unbundle By Name(w64) -> ("RT FIFOs--cluster.System Status RT FIFO"=w63:refnum<k33>, "Session in"=w62:refnum<k21>, "RT FIFOs--cluster.AIs RT FIFO out"=w60:refnum<k33>, "RT FIFOs--cluster.DIOs RT FIFO out"=w59:refnum<k33>)
            n137 = call "Get System Status.vi"("System Session"=w62) -> ("output cluster"=w61:T27)  [unwired: 8 in, 2 out]
            n138 = RT FIFO Read(0:w60) -> (9:w58:sgl[], 11:→"error out 2":errorcluster)  [unwired: 3 in, 3 out]
            n139 = RT FIFO Read(0:w59) -> (9:w57:bool[], 11:→"error out 3":errorcluster)  [unwired: 3 in, 3 out]
            n140 = RT FIFO Write(0:w63, 1:w61) -> ()  [unwired: 3 in, 4 out]
            n141 = call "Update AOs Values.vi"("AIs Values"=w58) -> ()  [unwired: 10 in, 1 out]
            n142 = call "Update DOs Values.vi"("DOs Values"=w57) -> ()  [unwired: 10 in, 1 out]
          }
          event User Event {
            n143 = event-data() -> ("RT FIFOs--cluster"=w67:T7)  [unwired: 1 in]
            n144 = call <vilib>:"Initialize Session.vi"() -> ("Session out"=w68:refnum<k21>)  [unwired: 10 in, 1 out]
            n145 = Bundle By Name(cluster=w69, "Session in"=w68, "RT FIFOs--cluster"=w67) -> (w66:T6)
          }
          event User Event {
            n146 = event-data() -> ()  [unwired: 1 in, 1 out]
            n147 = Unbundle By Name(w72) -> ("Session in"=w71:refnum<k21>)
            n148 = call-poly <vilib>:"Close.vi"("Session in"=w71) -> ()  [unwired: 10 in, 1 out]
          }
        }
        n149 = call-dynamic "Delacor_lib_QMH_Error Handler - Helper Loop.vi"("Error Debug"=w47, "error in"=w49, "Message Queue in"=w48) -> ()  [unwired: 7 in, 2 out]
      }
      n150 = Unregister For Events(event registration refnum=w35) -> ()  [unwired: 1 in, 1 out]
    }
    frame Error {
      # "Synchronize Caller Events.vi will inform Start Module.vi that the module has launched and will let the code calling Start Module.vi register for broadcasts and would permit the caller receive the broadcast that an error occurred at launch time."
      n151 = call-dynamic "Delacor_lib_QMH_Release Message Queue.vi"("error in"=w296, "Message Queue"=w289) -> ("error out"=w295:errorcluster)  [unwired: 9 in]
      n152 = call "Synchronize Caller Events.vi"("Singleton Module Admin in"=w290) -> ("error out"=w297:errorcluster)  [unwired: 9 in, 1 out]
      n153 = call "Module Name--constant.vi"() -> ("Module Name"=w293:string)  [unwired: 11 in]
      n154 = Format Into String(format string="An error occurred during initialization. %s is no longer running.", w293) -> (resulting string=w291:string)  [unwired: 2 in, 1 out]
      n155 = Merge Errors(w295, w297) -> (w298:errorcluster)
      n156 = call "Error Reported.vi"("Additional Information"=w291, "Error"=w298) -> ()  [unwired: 9 in, 1 out]
    }
  }
  n157 = Merge Errors(w28, w31) -> (w27:errorcluster)
  n158 = call "Close Module.vi"("error in"=w27, "Module Admin in"=w23) -> ("error out"=w29:errorcluster, "External Launch"=w17:bool, "Module Admin out"=w18:refnum<class "Delacor_lib_QMH_Module Admin.lvclass">)  [unwired: 7 in]
  n159 = Unregister For Events(event registration refnum=w22, error in=w29) -> (error out=w26:errorcluster)
  "error out" <- w26
  n160 = case "External Launch?" shown="True" w17 {
    tunnel: w26 -> [_ w299]
    frame False {
    }
    frame True {
      n161 = case shown="No Error" w299 {
        frame No Error {
          n162 = invoke on="Invoke Node" class="VI" method="FP.Close"() -> ()  [unwired: 3 in, 3 out]
        }
        frame Error {
          n163 = disable-structure shown="Default" {
            frame condition #0 (active) {
              n164 = invoke class="VI" method="FP.Open"("Activate"=TRUE ("Activate?")) -> ()  [unwired: 4 in, 5 out]
            }
            frame condition #1 {
              # "Don't show panel on error if running inside a built EXE."
            }
          }
        }
      }
    }
  }
  n165 = local write "Module Admin"(w18) -> ()
